vi "test_hashlib_sha256_pbkdf2.vi"() -> (3 "all_passed":bool)   [LabVIEW 2017]
uses:
  hashlib/rpacini_hashlib.lvlib
panel:
  out "sha256":string[](array[string])
  out "passed":bool[](array[boolean])
  in  "test_cases":T1(array[cluster])
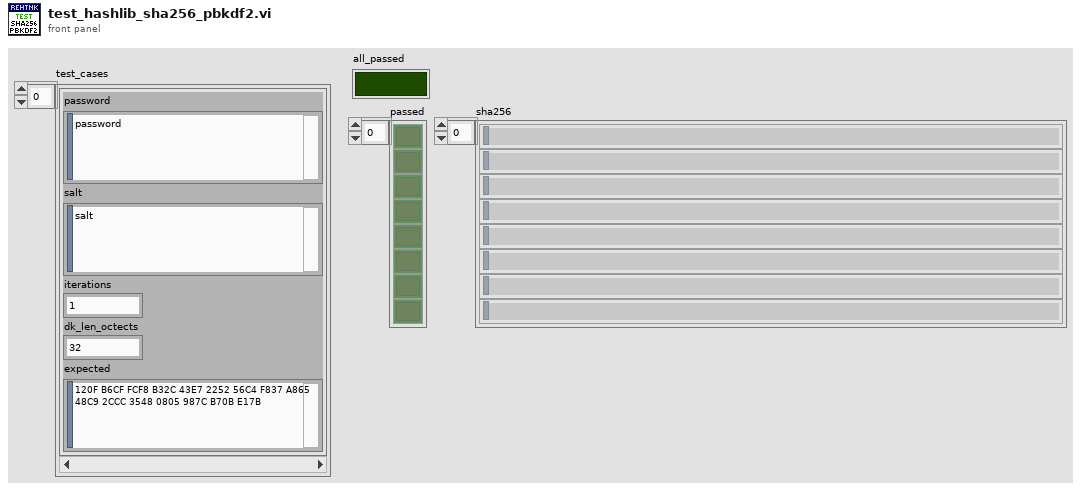
[diagram p1: front panel]
types:
  T1 = cluster{"password":string, "salt":string, "iterations":i32, "dk_len_octects":i32, "expected":string}[]
  T2 = cluster{"password":string, "salt":string, "iteration":i32, "dk_len_octects":i32, "expected":string}
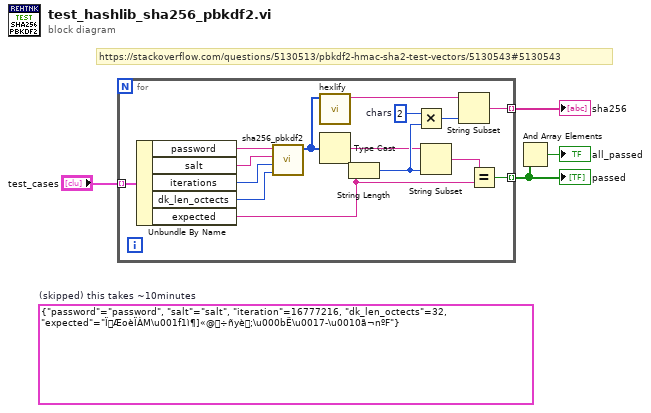
[diagram p0: block diagram]
diagram:
  (unwired) T2 {"password"="password", "salt"="salt", "iteration"=16777216, "dk_len_octects"=32, "expected"="ÏÆoèÏÀM\u001f1ì¶]«@÷ñyè;\u000bË\u0017­\u0010ã¬nºF"}  # (skipped) this takes ~10minutes
  # "https://stackoverflow.com/questions/5130513/pbkdf2-hmac-sha2-test-vectors/5130543#5130543"
  n1 = for {
    tunnel: "test_cases" -> [w19] mode=indexing
    tunnel: [w18] -> w3 mode=indexing
    tunnel: [w15] -> w1 mode=indexing
    w12 = 2  # chars
    n2 = Unbundle By Name(w19) -> ("password"=w9:string, "salt"=w8:string, "iterations"=w7:i32, "dk_len_octects"=w5:i32, "expected"=w17:string)
    n3 = call "sha256_pbkdf2.vi"("dkLen (32octets=sha256)"=w5, "iterations"=w7, "salt"=w8, "password"=w9) -> ("sha-256"=w6:u32[])  [unwired: 7 in]
    n4 = call "hexlify.vi"("sha256"=w6) -> ("hex (0-9a-f)"=w16:string)  [unwired: 10 in]
    n5 = Type Cast(x=w6) -> (*(type *) &x=w11:string)  [unwired: 1 in]
    n6 = String Length(string=w17) -> (length=w14:i32)
    n7 = Multiply(x=w12, y=w14) -> (x*y=w13:i32)
    n8 = String Subset(string=w11, length (rest)=w14) -> (substring=w10:string)  [unwired: 1 in]
    n9 = String Subset(string=w16, length (rest)=w13) -> (substring=w15:string)  [unwired: 1 in]
    n10 = Equal?(x=w10, y=w17) -> (x = y?=w18:bool)
  }
  "passed" <- w3
  "sha256" <- w1
  n11 = And Array Elements(Boolean array=w3) -> (logical AND=→"all_passed":bool)
